vi "Judge.vi"(11 "chess":bool[][](array[boolean])) -> (3 "Over?":bool)   [LabVIEW 2015]
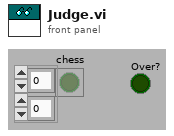
[diagram p1: front panel]
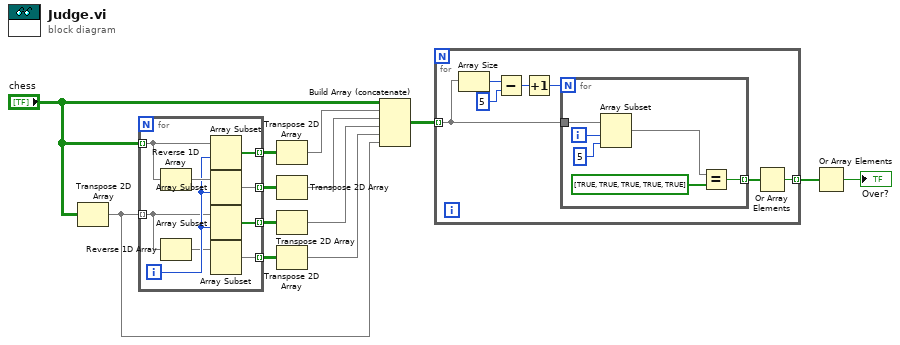
[diagram p0: block diagram]
diagram:
  n1 = Transpose 2D Array(2D array="chess") -> (transposed array=w2:bool[][])
  n2 = for {
    tunnel: "chess" -> [w20] mode=indexing
    tunnel: [w22] -> w13 mode=indexing
    tunnel: w2 -> [w17] mode=indexing
    tunnel: [w21] -> w8 mode=indexing
    tunnel: [w15] -> w7 mode=indexing
    tunnel: [w14] -> w6 mode=indexing
    i -> [w18]
    n3 = Reverse 1D Array(array=w20) -> (reversed array=w19:bool[])
    n4 = Reverse 1D Array(array=w17) -> (reversed array=w16:bool[])
    n5 = Array Subset(array=w20, index=w18) -> (w22:bool[])  [unwired: 1 in]
    n6 = Array Subset(array=w19, index=w18) -> (w15:bool[])  [unwired: 1 in]
    n7 = Array Subset(array=w17, index=w18) -> (w21:bool[])  [unwired: 1 in]
    n8 = Array Subset(array=w16) -> (w14:bool[])  [unwired: 2 in]
  }
  n9 = Transpose 2D Array(2D array=w13) -> (transposed array=w11:bool[][])
  n10 = Transpose 2D Array(2D array=w7) -> (transposed array=w5:bool[][])
  n11 = Transpose 2D Array(2D array=w8) -> (transposed array=w4:bool[][])
  n12 = Transpose 2D Array(2D array=w6) -> (transposed array=w3:bool[][])
  n13 = Build Array (concatenate)("chess", w11, w5, w4, w3, w2) -> (w10:bool[][])
  n14 = for {
    tunnel: w10 -> [w25] mode=indexing
    tunnel: [w23] -> w9 mode=indexing
    n15 = Array Size(array=w25) -> (size(s)=w29:i32)
    n16 = Subtract(x=w29, y=5) -> (x-y=w27:i32)
    n17 = Increment(x=w27) -> (x+1=w26:i32)
    n18 = for {
      N: w26 -> [_]
      tunnel: w25 -> [w35]
      tunnel: [w30] -> w24 mode=indexing
      i -> [w34]
      n19 = Array Subset(array=w35, index=w34, length=5) -> (w32:bool[])
      n20 = Equal?(x=w32, y=bool[] [TRUE, TRUE, TRUE, TRUE, TRUE]) -> (x = y?=w30:bool)
    }
    n21 = Or Array Elements(Boolean array=w24) -> (logical OR=w23:bool)
  }
  n22 = Or Array Elements(Boolean array=w9) -> (logical OR=→"Over?":bool)
